vi "SaveTRFFile.vi"(9 "Y":cdb[](array[numeric]), 10 "Header Info":T1, 11 "trf file in":path) -> (0 "error out":errorcluster, 3 "trf file out":path)   [LabVIEW 2022 SP3]
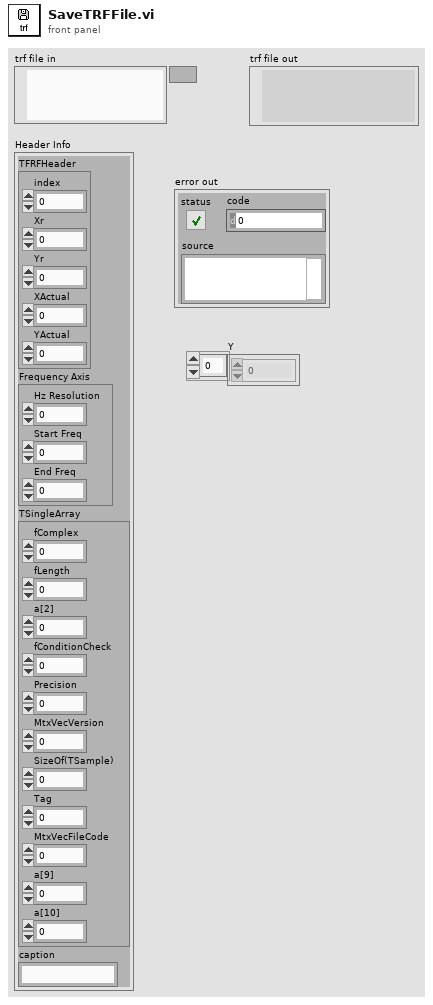
[diagram p1: front panel]
types:
  T1 = cluster{"TFRFHeader":cluster{"index":u32, "Xr":dbl, "Yr":dbl, "XActual":dbl, "YActual":dbl}, "Frequency Axis":cluster{"Hz Resolution":dbl, "Start Freq":dbl, "End Freq":dbl}, "TSingleArray":cluster{"fComplex":u32, "fLength":dbl, "a[2]":dbl, "fConditionCheck":dbl, "Precision":dbl, "MtxVecVersion":dbl, "SizeOf(TSample)":dbl, "Tag":dbl, "MtxVecFileCode":dbl, "a[9]":dbl, "a[10]":dbl}, "caption":string}
  T2 = enum16{"big-endian, network order", "native, host order", "little-endian"}
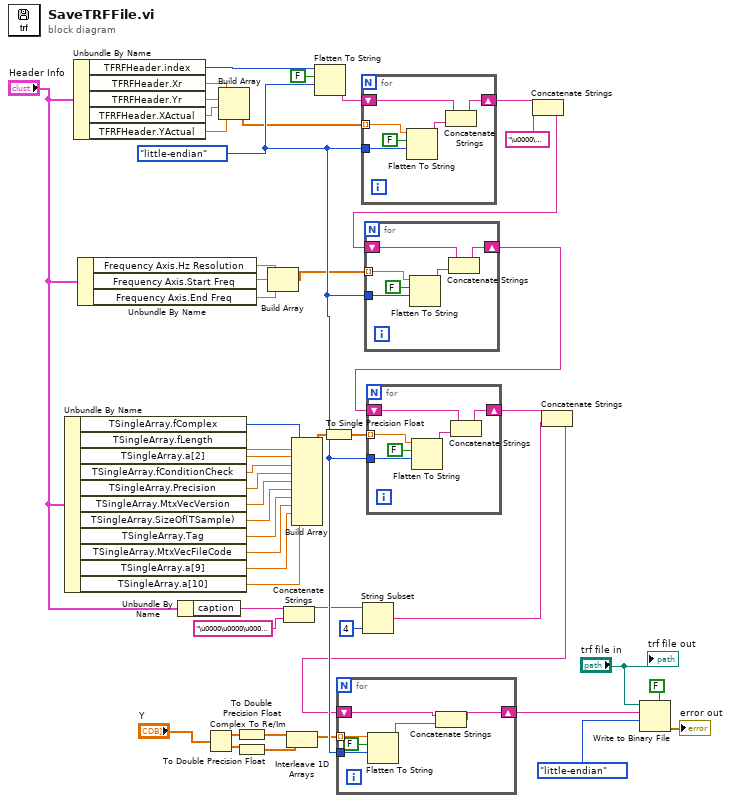
[diagram p0: block diagram]
diagram:
  w39 = T2."little-endian" ("byte order (0:big-endian, network order)")
  n1 = Unbundle By Name("Header Info") -> ("TSingleArray.fComplex"=w18:u32, "TSingleArray.fLength"=w19:dbl, "TSingleArray.a[2]"=w17:dbl, "TSingleArray.fConditionCheck"=w21:dbl, "TSingleArray.Precision"=w22:dbl, "TSingleArray.MtxVecVersion"=w23:dbl, "TSingleArray.SizeOf(TSample)"=w24:dbl, "TSingleArray.Tag"=w25:dbl, "TSingleArray.MtxVecFileCode"=w26:dbl, "TSingleArray.a[9]"=w27:dbl, "TSingleArray.a[10]"=w28:dbl)
  n2 = Unbundle By Name("Header Info") -> ("TFRFHeader.index"=w2:u32, "TFRFHeader.Xr"=w6:dbl, "TFRFHeader.Yr"=w3:dbl, "TFRFHeader.XActual"=w4:dbl, "TFRFHeader.YActual"=w5:dbl)
  n3 = Unbundle By Name("Header Info") -> ("Frequency Axis.Hz Resolution"=w12:dbl, "Frequency Axis.Start Freq"=w11:dbl, "Frequency Axis.End Freq"=w13:dbl)
  n4 = Unbundle By Name("Header Info") -> ("caption"=w31:string)
  n5 = Complex To Re/Im(x + iy="Y") -> (x=w33:dbl[], y=w34:dbl[])
  n6 = Build Array(w6, w3, w4, w5) -> (w7:dbl[])
  n7 = To Double Precision Float(number=w33) -> (double precision float=w35:dbl[])
  n8 = To Double Precision Float(number=w34) -> (double precision float=w36:dbl[])
  n9 = Build Array(w12, w11, w13) -> (w14:dbl[])
  n10 = Concatenate Strings(w31, "\u0000\u0000\u0000\u0000" ("string")) -> (w32:string)
  n11 = Interleave 1D Arrays(w35, w36) -> (w37:dbl[])
  n12 = Build Array(w18, w19, w17, w21, w22, w23, w24, w25, w26, w27, w28) -> (w16:dbl[])
  n13 = Flatten To String(anything=w2, prepend array or string size? (T)=FALSE, byte order (0:big-endian, network order)=w39) -> (data string=w8:string)  [unwired: 1 in, 2 out]
  n14 = To Single Precision Float(number=w16) -> (single precision float=w41:sgl[])
  n15 = for {
    tunnel: w39 -> [w54]
    tunnel: w7 -> [w53] mode=indexing
    shift-right: [w50] -> w9
    shift-left: w8 -> [w52]
    n16 = Flatten To String(anything=w53, prepend array or string size? (T)=FALSE, byte order (0:big-endian, network order)=w54) -> (data string=w51:string)  [unwired: 1 in, 2 out]
    n17 = Concatenate Strings(w52, w51) -> (w50:string)
  }
  n18 = String Subset(string=w32, length (rest)=4 ("length (rest)")) -> (substring=w42:string)  [unwired: 1 in]
  n19 = Concatenate Strings(w9, "\u0000\u0000" ("string")) -> (w15:string)
  n20 = for {
    tunnel: w39 -> [w60]
    tunnel: w14 -> [w59] mode=indexing
    shift-right: [w56] -> w20
    shift-left: w15 -> [w58]
    n21 = Flatten To String(anything=w59, prepend array or string size? (T)=FALSE, byte order (0:big-endian, network order)=w60) -> (data string=w57:string)  [unwired: 1 in, 2 out]
    n22 = Concatenate Strings(w58, w57) -> (w56:string)
  }
  n23 = for {
    tunnel: w39 -> [w66]
    tunnel: w41 -> [w65] mode=indexing
    shift-right: [w62] -> w29
    shift-left: w20 -> [w64]
    n24 = Flatten To String(anything=w65, prepend array or string size? (T)=FALSE, byte order (0:big-endian, network order)=w66) -> (data string=w63:string)  [unwired: 1 in, 2 out]
    n25 = Concatenate Strings(w64, w63) -> (w62:string)
  }
  n26 = Concatenate Strings(w29, w42) -> (w38:string)
  n27 = for {
    tunnel: w37 -> [w72] mode=indexing
    tunnel: w39 -> [w68]
    shift-right: [w69] -> w45
    shift-left: w38 -> [w71]
    n28 = Flatten To String(anything=w72, prepend array or string size? (T)=FALSE, byte order (0:big-endian, network order)=w68) -> (data string=w70:string)  [unwired: 1 in, 2 out]
    n29 = Concatenate Strings(w71, w70) -> (w69:string)
  }
  n30 = Write to Binary File(file (use dialog)="trf file in", data=w45, 5:FALSE ("prepend array or string size? (T)"), 9:T2."little-endian" ("byte order (0:big-endian, network order)")) -> (error out=→"error out":errorcluster)  [unwired: 2 in, 2 out]
  "trf file out" <- "trf file in"
